vi "New RegWriteExtLong Command.vi"(0 "RFFE RegWriteExt Command in":refnum<class "RFFE RegWriteExtLong Command.lvclass">, 1 "Alias":string, 5 "Slave Address":T3=12 format="%02x", 7 "Register Address":T2 format="%02x", 9 "Register Data":T1[](array[typedef]) format="%02x", 11 "error in (no error)":errorcluster) -> (4 "RFFE RegWriteExt Command out":refnum<class "RFFE RegWriteExtLong Command.lvclass">, 15 "error out":errorcluster)   [LabVIEW 2018, in "MIPI RFFE API.lvlib" / "RFFE RegWriteExtLong Command.lvclass"]
uses:
  RFFE RegWriteExtLong Command.lvclass
  C:/Users/semoore/Projects/mipi-rffe-labview-oop/RegWriteExt/RFFE RegWriteExt Command.lvclass
  Slave Address.ctl
  Register Address.ctl
  Register Data.ctl
  RegWriteExt/RFFE RegWriteExt Command.lvclass
  MIPI RFFE API.lvlib
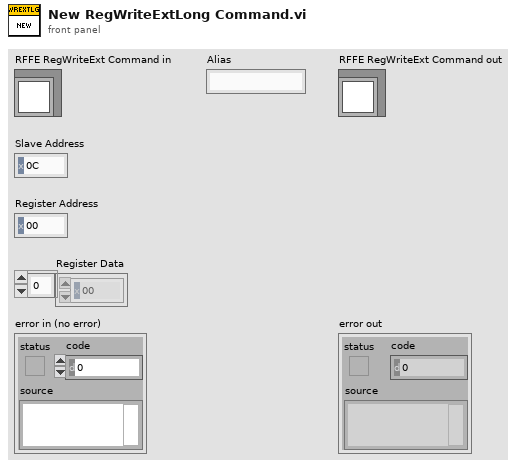
[diagram p1: front panel]
types:
  T1 = typedef "MIPI RFFE API.lvlib/Register Data.ctl" = u8
  T2 = typedef "MIPI RFFE API.lvlib/Register Address.ctl" = u16
  T3 = typedef "MIPI RFFE API.lvlib/Slave Address.ctl" = u8
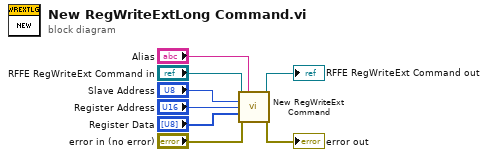
[diagram p0: block diagram]
diagram:
  n1 = call "New RegWriteExt Command.vi"("RFFE RegWriteExt Command in"="RFFE RegWriteExt Command in", "Alias"="Alias", "Slave Address"="Slave Address", "Register Address"="Register Address", "Register Data"="Register Data", "error in (no error)"="error in (no error)") -> ("RFFE RegWriteExt Command out"=→"RFFE RegWriteExt Command out":refnum<class "RFFE RegWriteExtLong Command.lvclass">, "error out"=→"error out":errorcluster)  [unwired: 8 in]
